vi "configure restart DIAdem.vi"(6 "Username (\"\")":string, 8 "error in (no error)":errorcluster) -> (0 "error out":errorcluster)   [LabVIEW 2011]
uses:
  server/DIAdem/lib/DIAdem Daemon Script Type.ctl
  server/DIAdem/lib/DIAdem Daemon Queue.ctl
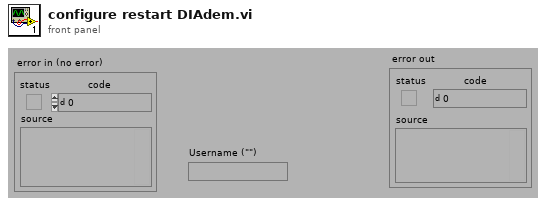
[diagram p1: front panel]
types:
  T1 = typedef "DIAdem Daemon Queue.ctl" = cluster{"Report Template TDM":path, "Report Processor VBS":path, "Report Path PDF":path, "Report Script Params":string, "Username":string, "Script Type":T2, "Report Query Params":string, "Client Machine":string, "Print on Client?":bool, "Response Queue Name":string, "Script Variables":string[], "Start Request Time":timestamp, "Wait?":bool}
  T2 = typedef "DIAdem Daemon Script Type.ctl" = enum16{"Report", "Query", "Script", "Datasheet", "Append", "Restart", "Stop"}
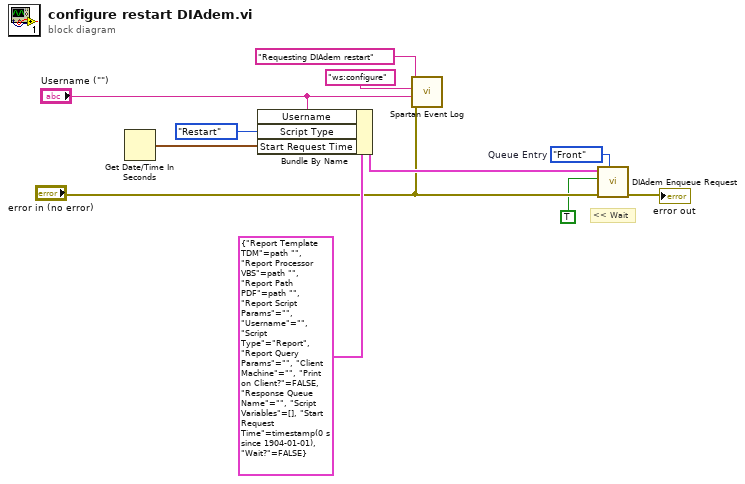
[diagram p0: block diagram]
diagram:
  w8 = enum16{"Front", "Back"}."Front"  # Queue Entry
  # "<< Wait"
  n1 = Get Date/Time In Seconds() -> (seconds since 1Jan1904=w9:timestamp)
  n2 = Bundle By Name(cluster=T1 {"Report Template TDM"=path "", "Report Processor VBS"=path "", "Report Path PDF"=path "", "Report Script Params"="", "Username"="", "Script Type"=enum."Report", "Report Query Params"="", "Client Machine"="", "Print on Client?"=FALSE, "Response Queue Name"="", "Script Variables"=[], "Start Request Time"=timestamp(0 s since 1904-01-01), "Wait?"=FALSE} ("DD_Report"), "Username"="Username (\"\")", "Script Type"=DIAdem_Daemon_Script_Type."Restart", "Start Request Time"=w9) -> (w10:T1)
  n3 = call "Spartan Event Log.vi"("error in (no error)"="error in (no error)", "username (\"\")"="Username (\"\")", "module (\"\")"="ws:configure" ("message (\"\")"), "message (\"\")"="Requesting DIAdem restart" ("message (\"\")")) -> ()  [unwired: 4 in, 1 out]
  n4 = call "DIAdem Enqueue Request.vi"("Queue Entry"=w8, "error in (no error)"="error in (no error)", "Wait for Completion? (f)"=TRUE, "DD_Report"=w10) -> ("error out"=→"error out":errorcluster)  [unwired: 1 in, 6 out]
